vi "Calibrate In Ear (FPL).vi"(11 "State":T2) -> (0 "error out":errorcluster)   [LabVIEW 2015]
uses:
  Utility VIs/Type Defs/Speaker ring.ctl
  Utility VIs/Buttons/KCheckmarkBoolean 2.ctl
  Cochlear Function Test Suite/LV Source/CFTS Main Panel SubVIs/CFTS-Experiment State.ctl
  FPL VIs/FPL-In Ear Parameters.ctl
  FPL VIs/FPL-Stimulus.ctl
  Utility VIs/Conversion VIs/Create Waveform Cluster (2D).vi
  Utility VIs/Math VIs/FFT x(t) to dB,Degrees (2D).vi
  Instance           1 24Saved   Calibrate In Ear .vi
panel:
  in  "Start":bool
  in  "Stop":bool
  in  "FPL":T1 caption="Compute FPL"
  in  "Speaker":T3
  in  "mic gain":dbl caption="Mic Gain (dB)"
  in  "Stimulus":T4={"Resolution (Hz)"=50.0, "Attenuation (dB)"=30.0, "Sampling rate (Hz)"=100000.0}
  out "Stimulus graph":cluster{i32, dbl, dbl[]}(graph)={0, 0.01, []}
  in  "Averages":i32=128
  in  "Tabs":enum32{"Live", "Data"}(tab)
  out "Mic signals":cluster{"offset":dbl, "dx":dbl, "Y":dbl[][]}(graph)
  out "Mic mag":cluster{"offset":dbl, "dx":dbl, "Y":dbl[][]}(graph)
  out "Acquired":i32=256
  in  "Clear":bool
  in  "Load":bool
  in  "Show all":bool
  out "ASTF":cluster{"Frequency":dbl[], "Frequency":dbl[]}[](graph)
  in  "Plot Max SPL":T1=TRUE
  in  "result":cluster{"Path":path, "error ":errorcluster}
  out "Path":path
  out "ASTF phase":cluster{"Frequency":dbl[], "Frequency":dbl[]}[](graph)
  out "Mic phase graph":cluster{"offset":dbl, "dx":dbl, "Y":dbl[][]}(graph)
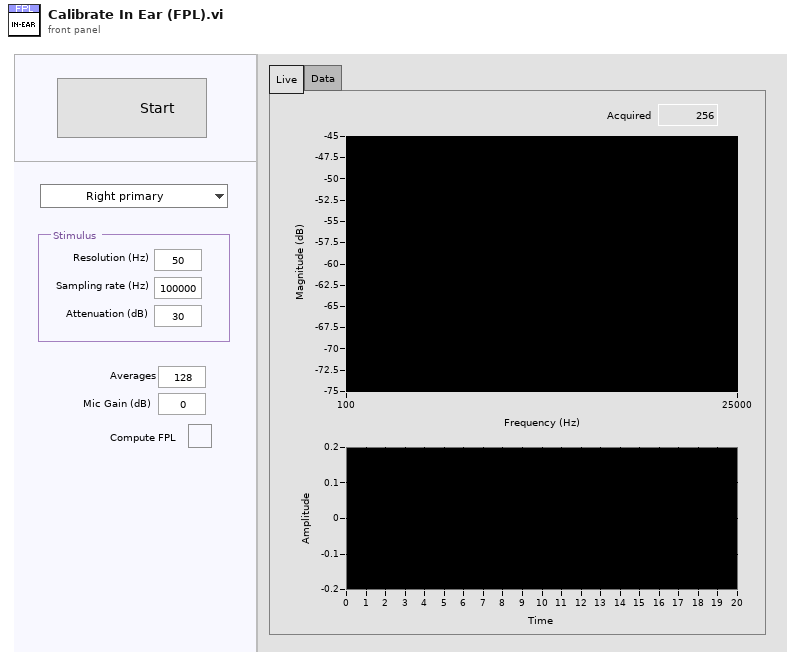
[diagram p1: front panel]
types:
  T1 = typedef "KCheckmarkBoolean 2.ctl" = bool
  T2 = typedef "CFTS-Experiment State.ctl" = cluster{"Experimenter":string, "Number":u32, "Right":string, "Left":string, "Data Folder":path, "State File":path, "Version Info":string, "End Exposure Time":dbl, "Exposure Duration":string, "Run #":cluster{"CAP":i16, "ABR":i16, "DP":i16, "VsEP":i16, "MeasSeq":i16, "SubSeq":i16, "SFOAE":i16}}
  T3 = typedef "Speaker ring.ctl" = enum16{"Right primary", "Right secondary", "Left primary", "Left secondary"}
  T4 = cluster{"Resolution (Hz)":dbl, "Attenuation (dB)":dbl, "Sampling rate (Hz)":dbl}
  T5 = typedef "FPL-In Ear Parameters.ctl" = cluster{"Speaker":T3, "Stimulus":T6, "Averages":i32, "Left gain":dbl, "Right gain":dbl, "plot max":bool, "FPL":bool}
  T6 = typedef "FPL-Stimulus.ctl" = cluster{"Resol (Hz)":dbl, "Atten (dB)":dbl, "Fs (Hz)":dbl}
  T7 = typedef "Cal Stimulus.ctl" = cluster{"Min Freq (Hz)":dbl, "Max Freq (Hz)":dbl, "Freq Step (Hz)":dbl, "Waveform":enum16{"Chirp", "Weighted"}, "Attenuation (dB)":dbl, "Sample Rate (Hz)":dbl}
  T8 = cluster{"path out":path, "error out":errorcluster}
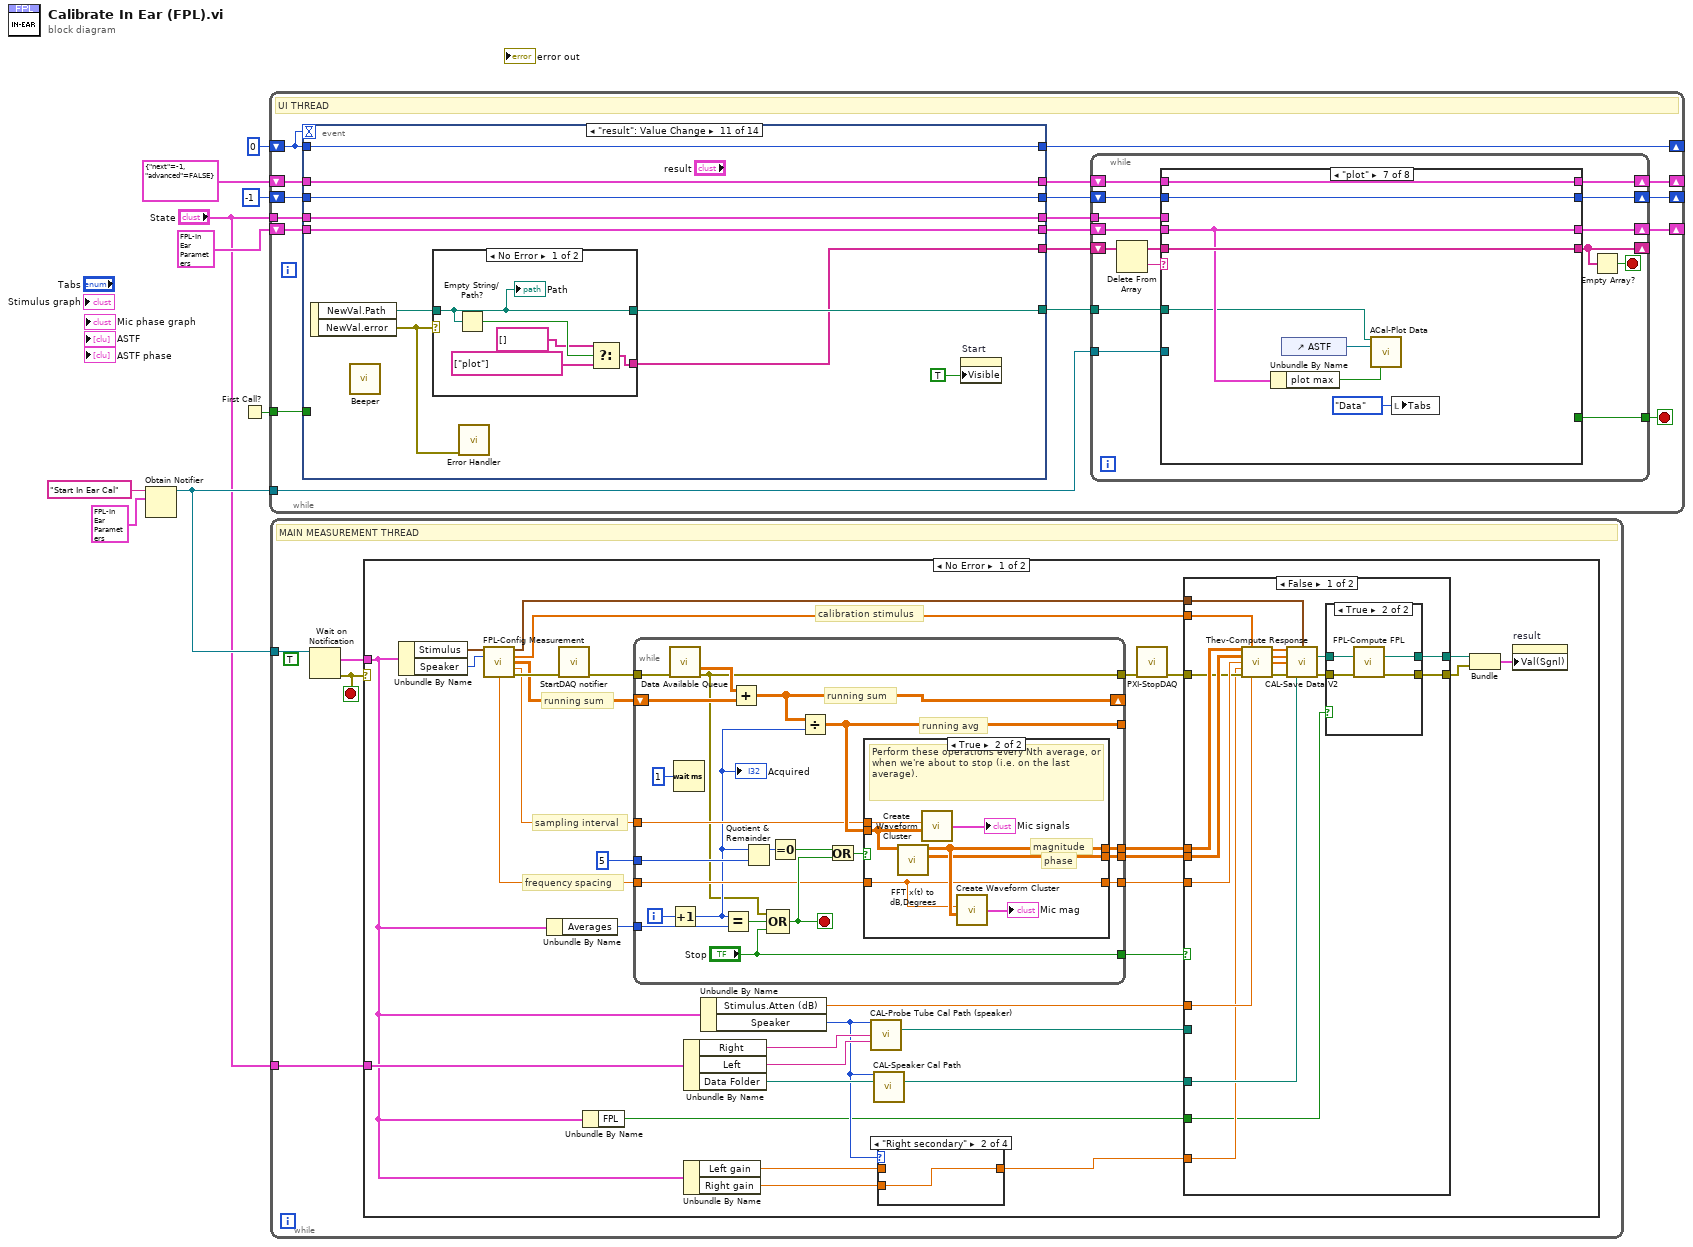
[diagram p0: block diagram]
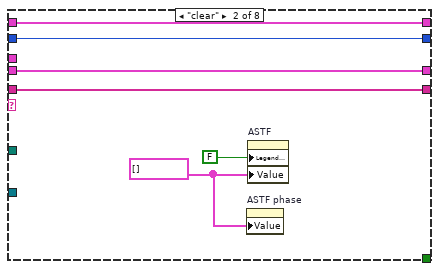
[diagram p10: hidden frame]
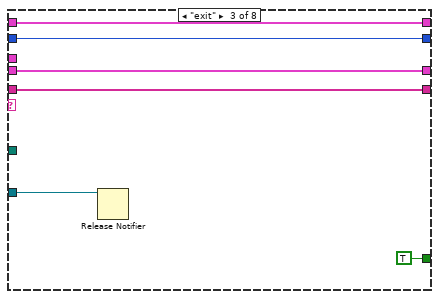
[diagram p11: hidden frame]
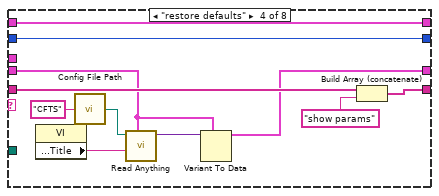
[diagram p12: hidden frame]
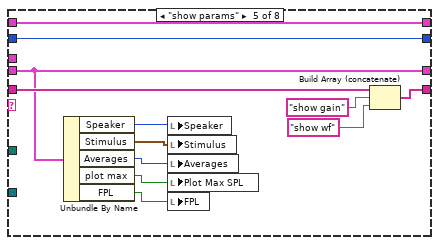
[diagram p13: hidden frame]
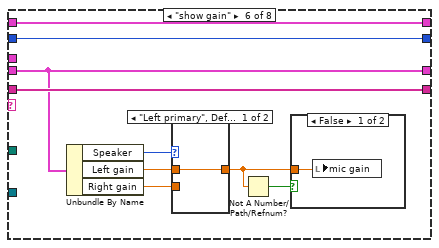
[diagram p14: hidden frame]
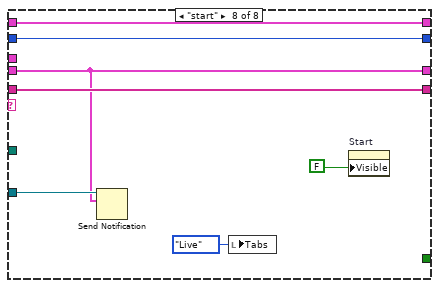
[diagram p17: hidden frame]
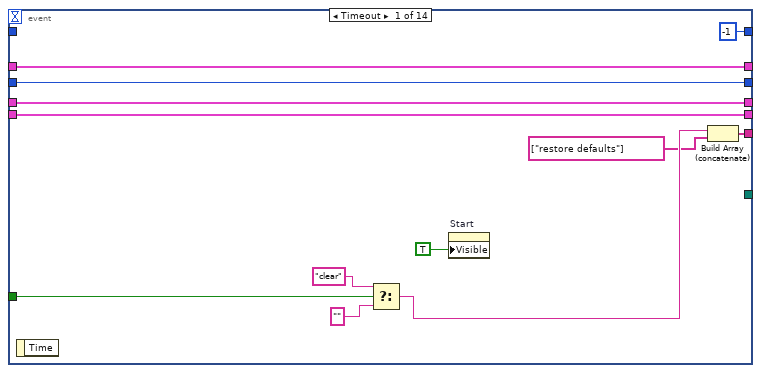
[diagram p18: hidden frame]
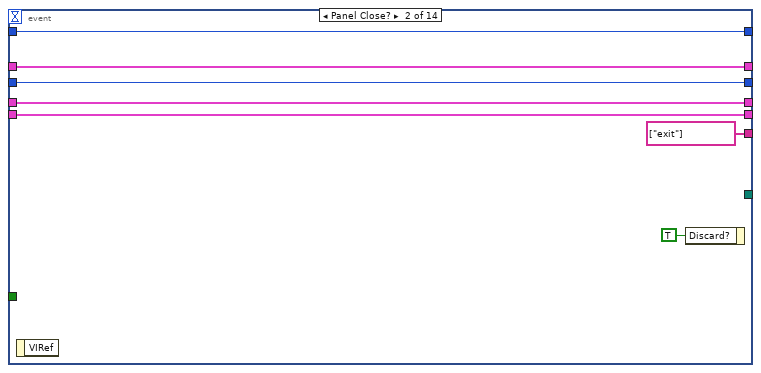
[diagram p19: hidden frame]
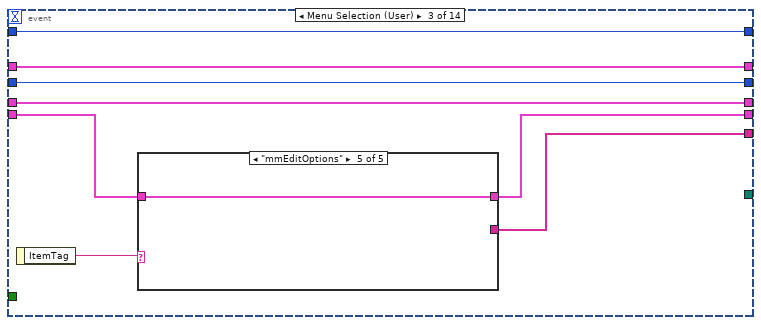
[diagram p20: hidden frame]
diagram:
  n1 = Obtain Notifier(name (unnamed)="Start In Ear Cal", notification data type=T5 {"Speaker"=enum."Right primary", "Stimulus"={"Resol (Hz)"=50.0, "Atten (dB)"=50000.0, "Fs (Hz)"=50.0}, "Averages"=512, "Left gain"=40.0, "Right gain"=40.0, "plot max"=TRUE, "FPL"=FALSE} ("Params")) -> (notifier out=w9:refnum<notifier>)  [unwired: 2 in, 2 out]
  n2 = First Call?() -> (First Call?: T/F=w1:bool)
  n3 = while {
    tunnel: w9 -> [w16]
    shift-right: [w25] -> _
    shift-left: 0 -> [w26]
    shift-right: [w19] -> _
    shift-left: -1 -> [w27]
    tunnel: "State" -> [w24]
    shift-right: [w20] -> _
    shift-left: T5 {"Speaker"=enum."Right primary", "Stimulus"={"Resol (Hz)"=50.0, "Atten (dB)"=50000.0, "Fs (Hz)"=50.0}, "Averages"=512, "Left gain"=40.0, "Right gain"=40.0, "plot max"=TRUE, "FPL"=TRUE} ("Params") -> [w23]
    shift-right: [w11] -> _
    shift-left: cluster{"next":i32, "advanced":bool} {"next"=-1, "advanced"=FALSE} -> [w13]
    tunnel: w1 -> [w10]
    stop <- w17 stop-if-true
    # "UI THREAD"
    n4 = event shown="[10] \"result\": Value Change" {
      selector: _ -> [_ _ _ _ _ _ _ _ _ _ _ _ _ _]
      dyn-events: _ -> [_ _ _ _ _ _ _ _ _ _ _ _ _ _]
      timeout: w26 -> [_ _ _ _ _ _ _ _ _ _ _ _ _ _]
      tunnel: w27 -> [w119 w126 w135 w154 w162 w165 w172 w180 w192 w205 w227 w239 w246 w261]
      tunnel: [w119 w126 w135 w154 w162 w165 w172 w180 w192 w205 w227 w239 w246 w261] -> w22
      tunnel: w26 -> [_ w125 w134 w153 w161 w170 w177 w184 w191 w204 w226 w238 w245 w259]
      tunnel: [-1 w125 w134 w153 w161 w170 w177 w184 w191 w204 w226 w238 w245 w259] -> w25
      tunnel: w24 -> [w115 w122 w129 w152 w156 w168 w175 w182 w187 w202 w224 w235 w243 w258]
      tunnel: w23 -> [w117 w124 w132 w151 w160 w169 w176 w183 w189 w203 w225 w237 w244 w257]
      tunnel: [w117 w124 w131 w151 w158 w167 w174 w181 w188 w201 w225 w237 w244 w257] -> w21
      tunnel: [w114 string[] ["exit"] w130 string[] ["start"] string[] ["show gain"] string[] ["show wf"] _ _ _ _ w219 string[] ["clear"] w241 _] -> w18
      tunnel: [w115 w122 w129 w152 w156 w168 w175 w182 w187 w202 w224 w235 w243 w258] -> w15
      tunnel: [_ _ _ _ _ _ _ _ _ _ w222 _ w242 _] -> w14
      tunnel: w13 -> [w112 w121 w128 w150 w155 w164 w171 w179 w185 w199 w221 w234 w240 w255]
      tunnel: [w112 w121 w128 w150 w155 w164 w171 w179 w185 w199 w221 w234 w240 w255] -> w12
      tunnel: w10 -> [w111 _ _ _ _ _ _ _ _ _ _ _ _ _]
      event Timeout {
        n5 = event-data() -> ()  [unwired: 1 in, 1 out]
        n6 = Select(t="clear", s=w111, f="") -> (s? t:f=w116:string)
        n7 = property on="Start" class="Bool"("Visible"=TRUE) -> ()  [unwired: 2 in, 2 out]
        n8 = Build Array (concatenate)(w116, string[] ["restore defaults"]) -> (w114:string[])
      }
      event Panel Close? {
        n9 = event-data() -> ()  [unwired: 1 in, 1 out]
        n10 = event-data("Discard?"=TRUE) -> ()  [unwired: 1 in, 1 out]
      }
      event Menu Selection (User) {
        n11 = event-data() -> ("ItemTag"=w133:string)  [unwired: 1 in]
        n12 = case shown="\"mmEditOptions\"" w133 {
          tunnel: w132 -> [w136 w138 w141 w147 w148]
          tunnel: [w136 w138 w141 w147 w148] -> w131
          tunnel: [_ string[] ["restore defaults"] _ string[] ["exit"] _] -> w130
          frame "", Default {
          }
          frame "mmFileRestore" {
          }
          frame "mmFileSave" {
            n13 = property class="VI"() -> ("Front Panel.Title"=w140:string)  [unwired: 2 in, 2 out]
            n14 = call "Config File Path.vi"("AppName"="CFTS") -> ("Default config file name"=w142:path)
            n15 = call "Write Anything.vi"("Section Name (Name of \"Anything\")"=w140, "Anything"=w141, "Path (dialog)"=w142) -> ("Error Out"=w139:errorcluster)  [unwired: 7 in, 1 out]
            n16 = case shown="Error" w139 {
              selector: w139 -> [_ w145]
              frame No Error {
                n17 = One Button Dialog(message="Defaults saved.") -> ()  [unwired: 1 in, 1 out]
              }
              frame Error {
                n18 = call "Error Handler.vi"("error in (no error)"=w145) -> ()  [unwired: 13 in, 2 out]
              }
            }
          }
          frame "mmFileExit" {
          }
          frame "mmEditOptions" {
          }
        }
      }
      event "Start": Value Change {
        n19 = event-data() -> ()  [unwired: 1 in, 1 out]
      }
      event Value Change {
        n20 = event-data() -> ("NewVal"=w157:T3)  [unwired: 1 in]
        n21 = Bundle By Name(cluster=w160, "Speaker"=w157) -> (w158:T5)
      }
      event "Stimulus": Value Change {
        n22 = event-data() -> ()  [unwired: 1 in, 1 out]
        n23 = Bundle By Name(cluster=w169, "Stimulus"="Stimulus") -> (w167:T5)
      }
      event "Averages": Value Change {
        n24 = event-data() -> ()  [unwired: 1 in, 1 out]
        n25 = Bundle By Name(cluster=w176, "Averages"="Averages") -> (w174:T5)
      }
      event Value Change {
        n26 = event-data() -> ()  [unwired: 1 in, 1 out]
        n27 = Bundle By Name(cluster=w183, "FPL"="FPL") -> (w181:T5)
      }
      event "mic gain": Value Change {
        n28 = event-data() -> ()  [unwired: 1 in, 1 out]
        n29 = Unbundle By Name(w189) -> ("Speaker"=w190:T3)
        n30 = case shown="\"Right primary\", \"Right secondary\"" w190 {
          tunnel: w189 -> [w195 w198]
          tunnel: [w194 w197] -> w188
          tunnel: "mic gain" -> [w193 w196]
          frame "Left primary", Default {
            n31 = Bundle By Name(cluster=w195, "Left gain"=w193) -> (w194:T5)
          }
          frame "Right primary", "Right secondary" {
            n32 = Bundle By Name(cluster=w198, "Right gain"=w196) -> (w197:T5)
          }
        }
      }
      event Value Change {
        # "Clear the plot because the scaling is no longer consistent with the option. We haven't retained a list of displayed data files, so we can't restore them with the proper scaling. The best we can do (without more serious revision) is to reload the last saved calibration file."
        n33 = event-data() -> ("NewVal"=w210:T1)  [unwired: 1 in]
        n34 = control-ref of="ASTF"() -> (w208:refnum<vi>)
        n35 = property class="XYGraph (strict)"(reference=w208, "Value"=cluster{"Frequency":dbl[], "Frequency":dbl[]}[] []) -> (reference out=w206:refnum<vi>, error out=w209:errorcluster)  [unwired: 1 in]
        n36 = Bundle By Name(cluster=w203, "plot max"="Plot Max SPL") -> (w201:T5)
        n37 = local read "Path"() -> (w212:path)
        n38 = call "FileIO-File or Folder Exists.vi"("error in (no error)"=w209, "path"=w212) -> ("Directory?"=w213:bool, "dup path"=w211:path)  [unwired: 6 in, 2 out]
        n39 = case shown="True" w213 {
          tunnel: w206 -> [_ w216]
          tunnel: w210 -> [_ w214]
          tunnel: w211 -> [_ w217]
          frame False {
          }
          frame True {
            n40 = call "ACal-Plot Data.vi"("Path"=w217, "Mag graph"=w216, "Plot max"=w214) -> ("error out"=w215:errorcluster)  [unwired: 11 in, 1 out]
            n41 = call <vilib>:"Simple Error Handler.vi"("error in (no error)"=w215) -> ()  [unwired: 4 in, 5 out]
          }
        }
      }
      event "result": Value Change {
        n42 = event-data() -> ("NewVal.Path"=w223:path, "NewVal.error"=w218:errorcluster)  [unwired: 1 in]
        n43 = call "Beeper.vi"() -> ()  [unwired: 5 in, 1 out]
        n44 = case shown="No Error" w218 {
          selector: w218 -> [_ w233]
          tunnel: w223 -> [w232 _]
          tunnel: [w232 _] -> w222
          tunnel: [w229 _] -> w219
          frame No Error {
            n45 = Empty String/Path?(string/path=w232) -> (empty?=w231:bool)
            n46 = Select(t=string[] [], s=w231, f=string[] ["plot"]) -> (s? t:f=w229:string[])
            "Path" <- w232
          }
          frame Error {
            n47 = call "Error Handler.vi"("error in (no error)"=w233) -> ()  [unwired: 13 in, 2 out]
          }
        }
        n48 = call "Error Handler.vi"("error in (no error)"=w218) -> ()  [unwired: 13 in, 2 out]
        n49 = property on="Start" class="Bool"("Visible"=TRUE) -> ()  [unwired: 2 in, 2 out]
      }
      event "Clear": Value Change {
        n50 = event-data() -> ()  [unwired: 1 in, 1 out]
      }
      event "Load": Value Change {
        n51 = event-data() -> ()  [unwired: 1 in, 1 out]
        n52 = Unbundle By Name(w243) -> ("Data Folder"=w247:path)
        n53 = call "File Dialog"("start path"=w247, "pattern (all files)"="*.calib", "pattern label"="Calibration files") -> ("selected path"=w252:path, "cancelled"=w251:bool, "error out"=w250:errorcluster)  [unwired: 9 in, 1 out]
        n54 = case shown="False" w251 {
          tunnel: w252 -> [w254 _]
          tunnel: w250 -> [_ _]
          tunnel: [w254 _] -> w242
          tunnel: [string[] ["plot"] _] -> w241
          frame False {
          }
          frame True {
          }
        }
      }
      event "Show all": Value Change {
        n55 = event-data() -> ()  [unwired: 1 in, 1 out]
        n56 = Unbundle By Name(w257) -> ("plot max"=w256:bool)
        n57 = Unbundle By Name(w258) -> ("Data Folder"=w262:path)
        n58 = control-ref of="ASTF"() -> (w260:refnum<vi>)
        n59 = call "CAL-Show all.vi"("Path"=w262, "Mag graph"=w260, "Plot Max SPL"=w256) -> ("error out"=w263:errorcluster)  [unwired: 11 in, 1 out]
        n60 = call "Error Handler.vi"("error in (no error)"=w263) -> ()  [unwired: 13 in, 2 out]
      }
    }
    n61 = while {
      shift-right: [w40] -> w20
      shift-left: w21 -> [w41]
      shift-right: [w39] -> w19
      shift-left: w22 -> [w42]
      shift-right: [w35] -> _
      shift-left: w18 -> [w37]
      tunnel: w16 -> [w33]
      tunnel: [w32] -> w17
      tunnel: w15 -> [w31]
      tunnel: w14 -> [w30]
      shift-right: [w29] -> w11
      shift-left: w12 -> [w28]
      stop <- w34 stop-if-true
      n62 = Delete From Array(array=w37) -> (deleted portion=w36:string, array with subset deleted=w38:string[])  [unwired: 2 in]
      n63 = case shown="\"plot\"" w36 {
        tunnel: w42 -> [w46 w52 w58 w69 w81 w90 w101 w108]
        tunnel: [w46 w52 w58 w69 w81 w90 w101 w108] -> w39
        tunnel: w41 -> [w45 w51 w57 w65 w79 w88 w99 w104]
        tunnel: [w45 w51 w57 w64 w79 w88 w99 w104] -> w40
        tunnel: w38 -> [w44 w50 w56 w68 w80 w89 w100 w105]
        tunnel: [w44 w50 w56 w63 w74 w89 w100 w105] -> w35
        tunnel: w33 -> [_ _ w55 _ _ _ _ w106]
        tunnel: [_ _ TRUE _ _ _ _ _] -> w32
        tunnel: w31 -> [_ _ _ _ _ _ _ _]
        tunnel: w30 -> [_ _ _ _ _ _ w96 _]
        tunnel: [w43 w47 w53 w59 w72 w82 w95 w107] -> w29
        tunnel: w28 -> [w43 w47 w53 w59 w72 w82 w95 w107]
        frame "", Default {
        }
        frame "clear" {
          w49 = cluster{"Frequency":dbl[], "Frequency":dbl[]}[] [] ("ASTF mag")
          n64 = property on="ASTF phase" class="XYGraph (strict)"("Value"=w49) -> ()  [unwired: 2 in, 2 out]
          n65 = property on="ASTF" class="XYGraph (strict)"("Legend Visible"=FALSE ("Legend:Visible"), "Value"=w49) -> ()  [unwired: 2 in, 2 out]
        }
        frame "exit" {
          n66 = Release Notifier(notifier=w55) -> ()  [unwired: 2 in, 3 out]
        }
        frame "restore defaults" {
          n67 = property class="VI"() -> ("Front Panel.Title"=w61:string)  [unwired: 2 in, 2 out]
          n68 = call "Config File Path.vi"("AppName"="CFTS") -> ("Default config file name"=w60:path)
          n69 = call "Read Anything.vi"("Type of Anything"=w65, "Section Name (Name of \"Type of Anything\")"=w61, "Path (dialog)"=w60) -> ("Anything"=w66:variant)  [unwired: 6 in, 2 out]
          n70 = Variant To Data(type=w65, Variant=w66) -> (data=w64:T5)  [unwired: 1 in, 1 out]
          n71 = Build Array (concatenate)(w68, "show params") -> (w63:string[])
        }
        frame "show params" {
          n72 = Unbundle By Name(w79) -> ("Speaker"=w78:T3, "Stimulus"=w77:T6, "Averages"=w76:i32, "plot max"=w75:bool, "FPL"=w70:bool)
          n73 = local write "Speaker"(w78) -> ()
          n74 = local write "Stimulus"(w77) -> ()
          n75 = local write "Averages"(w76) -> ()
          n76 = local write "Plot Max SPL"(w75) -> ()
          n77 = local write "FPL"(w70) -> ()
          n78 = Build Array (concatenate)(w80, "show gain", "show wf") -> (w74:string[])
        }
        frame "show gain" {
          n79 = Unbundle By Name(w88) -> ("Speaker"=w85:T3, "Left gain"=w84:dbl, "Right gain"=w83:dbl)
          n80 = case shown="\"Left primary\", Default" w85 {
            tunnel: w84 -> [w92 _]
            tunnel: w83 -> [_ w93]
            tunnel: [w92 w93] -> w87
            frame "Left primary", Default {
            }
            frame "Right primary", "Right secondary" {
            }
          }
          n81 = Not A Number/Path/Refnum?(number/path/refnum=w87) -> (NaN/Path/Refnum?=w86:bool)
          n82 = case shown="False" w86 {
            tunnel: w87 -> [w91 _]
            frame False {
              n83 = local write "mic gain"(w91) -> ()
            }
            frame True {
            }
          }
        }
        frame "plot" {
          n84 = Unbundle By Name(w99) -> ("plot max"=w98:bool)
          n85 = control-ref of="ASTF"() -> (w97:refnum<vi>)
          n86 = call "ACal-Plot Data.vi"("Path"=w96, "Mag graph"=w97, "Plot max"=w98) -> ()  [unwired: 11 in, 2 out]
          n87 = local write "Tabs"(enum32{"Live", "Data"}."Data" ("Tabs")) -> ()
        }
        frame "start" {
          n88 = Send Notification(notification=w104, notifier=w106) -> ()  [unwired: 1 in, 2 out]
          n89 = local write "Tabs"(enum32{"Live", "Data"}."Live" ("Tabs")) -> ()
          n90 = property on="Start" class="Bool"("Visible"=FALSE) -> ()  [unwired: 2 in, 2 out]
        }
      }
      n91 = Empty Array?(array=w35) -> (empty?=w34:bool)
    }
  }
  n92 = while {
    tunnel: w9 -> [w267]
    tunnel: "State" -> [w265]
    stop <- w266 stop-if-true
    (unwired) TRUE
    # "MAIN MEASUREMENT THREAD"
    n93 = Wait on Notification(notifier=w267) -> (notification=w264:T5, error out=w266:errorcluster)  [unwired: 3 in, 2 out]
    n94 = case shown="No Error" w266 {
      tunnel: w265 -> [w282 _]
      tunnel: w264 -> [w270 _]
      frame No Error {
        # "calibration stimulus"
        # "frequency spacing"
        # "sampling interval"
        # "running sum"
        n95 = Unbundle By Name(w270) -> ("Stimulus"=w268:T6, "Speaker"=w281:T3)
        n96 = call "FPL-Config Measurement.vi"("Chirp spec in"=w268, "Speaker"=w281) -> ("Cal Stimulus"=w284:T7, "Stimulus"=w293:dbl[], "Mic Avg"=w299:dbl[][], "dt (ms)"=w297:dbl, "df (Hz)"=w298:dbl, "error out"=w300:errorcluster)  [unwired: 8 in]
        n97 = Unbundle By Name(w270) -> ("Averages"=w280:i32)
        n98 = call "StartDAQ notifier.vi"("error in (no error)"=w300) -> ("error out"=w292:errorcluster)  [unwired: 6 in]
        n99 = Unbundle By Name(w270) -> ("FPL"=w269:bool)
        n100 = while {
          tunnel: w292 -> [w351]
          tunnel: [w331] -> w291
          tunnel: w280 -> [w348]
          shift-right: [w346] -> _
          shift-left: w299 -> [w347]
          tunnel: [w345] -> _
          tunnel: 5 -> [w344]
          tunnel: w298 -> [w339]
          tunnel: [w338] -> w296
          tunnel: [w337] -> w295
          tunnel: w297 -> [w336]
          tunnel: [w335] -> w294
          tunnel: ["Stop"] -> w278
          i -> [w350]
          stop <- w340 stop-if-true
          # "running avg"
          # "running sum"
          n101 = call "Data Available Queue.vi"("error in (no error)"=w351) -> ("AI Waveforms"=w333:dbl[][], "error out"=w331:errorcluster)  [unwired: 10 in, 3 out]
          n102 = Increment(x=w350) -> (x+1=w334:i32)
          "Acquired" <- w334
          n103 = Wait (ms)(milliseconds to wait=u32 1) -> ()  [unwired: 1 out]
          n104 = Equal?(x=w334, y=w348) -> (x = y?=w349:bool)
          n105 = Add(x=w333, y=w347) -> (x+y=w346:dbl[][])
          n106 = Quotient & Remainder(x=w334, y=w344) -> (x-y*floor(x/y)=w343:i32)  [unwired: 1 out]
          n107 = Compound Arithmetic op=OR(w331, w349, "Stop") -> (w340:bool)
          n108 = Equal To 0?(x=w343) -> (x = 0?=w341:bool)
          n109 = Divide(x=w346, y=w334) -> (x/y=w345:dbl[][])
          n110 = Or(x=w341, y=w340) -> (x .or. y?=w342:bool)
          n111 = case shown="True" w342 {
            tunnel: w345 -> [_ w355]
            tunnel: w339 -> [_ w352]
            tunnel: [_ w357] -> w338
            tunnel: [_ w356] -> w337
            tunnel: w336 -> [_ w354]
            tunnel: [_ w352] -> w335
            frame False {
            }
            frame True {
              # "phase"
              # "magnitude"
              # "Perform these operations every Nth average, or when we're about to stop (i.e. on the last average)."
              n112 = call-poly "FFT x(t) to dB,Degrees.vi"("X(t)"=w355) -> ("+Freq Phase of FFT (degrees)"=w356:dbl[][], "+Freq. Mag of FFT (dB rms)"=w357:dbl[][])  [unwired: 9 in]
              n113 = call-poly "Create Waveform Cluster.vi"("dx"=w354, "Array"=w355) -> ("waveform cluster"=→"Mic signals":cluster{"offset":dbl, "dx":dbl, "Y":dbl[][]})  [unwired: 3 in]
              n114 = call-poly "Create Waveform Cluster.vi"("dx"=w352, "Array"=w357) -> ("waveform cluster"=→"Mic mag":cluster{"offset":dbl, "dx":dbl, "Y":dbl[][]})  [unwired: 3 in]
            }
          }
        }
        n115 = Unbundle By Name(w282) -> ("Right"=w289:string, "Left"=w288:string, "Data Folder"=w287:path)
        n116 = Unbundle By Name(w270) -> ("Left gain"=w276:dbl, "Right gain"=w274:dbl)
        n117 = Unbundle By Name(w270) -> ("Stimulus.Atten (dB)"=w279:dbl, "Speaker"=w277:T3)
        n118 = call "CAL-Probe Tube Cal Path (speaker).vi"("Speaker"=w277, "Right"=w289, "Left"=w288) -> ("Probe Tube Cal Path"=w286:path)  [unwired: 11 in, 1 out]
        n119 = call "CAL-Speaker Cal Path.vi"("Speaker"=w277, "Data Folder"=w287) -> ("Cal Path"=w283:path)  [unwired: 12 in, 1 out]
        n120 = case shown="\"Right secondary\"" w277 {
          tunnel: w276 -> [_ _ w303 w304]
          tunnel: [w301 w302 w303 w304] -> w275
          tunnel: w274 -> [w301 w302 _ _]
          frame "Right primary", Default {
          }
          frame "Right secondary" {
          }
          frame "Left secondary" {
          }
          frame "Left primary" {
          }
        }
        n121 = call "PXI-StopDAQ.vi"("error in (no error)"=w291) -> ("error out"=w285:errorcluster)  [unwired: 6 in]
        n122 = case shown="False" w278 {
          tunnel: w296 -> [w322 _]
          tunnel: w295 -> [w321 _]
          tunnel: w294 -> [w320 _]
          tunnel: w293 -> [w319 _]
          tunnel: w286 -> [_ _]
          tunnel: w285 -> [w318 w329]
          tunnel: w284 -> [w310 _]
          tunnel: w283 -> [w317 _]
          tunnel: w279 -> [w316 _]
          tunnel: [w306 w329] -> w272
          tunnel: [w307 _] -> w273
          tunnel: w275 -> [w315 _]
          tunnel: w269 -> [w305 _]
          frame False {
            n123 = call "Thev-Compute Response.vi"("Mag"=w322, "Stimulus"=w319, "Phase"=w321, "df (Hz)"=w320, "Probe Mic Gain (dB)"=w315, "error in (no error)"=w318, "Attenuation (dB)"=w316) -> ("ASTF Mag"=w311:dbl[], "ASTF Phase"=w312:dbl[], "Frequency"=w313:dbl[], "error out"=w314:errorcluster)  [unwired: 5 in]
            n124 = call "CAL-Save Data V2.vi"("Mag"=w311, "Cal Stimulus"=w310, "Phase"=w312, "Frequency"=w313, "error in (no error)"=w314, "path"=w317) -> ("new file path"=w308:path, "error out"=w309:errorcluster)  [unwired: 8 in]
            n125 = case shown="True" w305 {
              tunnel: w309 -> [w323 w328]
              tunnel: w308 -> [w324 w327]
              tunnel: [w324 w326] -> w307
              tunnel: [w323 w325] -> w306
              frame False {
              }
              frame True {
                n126 = call "FPL-Compute FPL.vi"("path in"=w327, "error in (no error)"=w328) -> ("path out"=w326:path, "error out"=w325:errorcluster)  [unwired: 12 in]
              }
            }
          }
          frame True {
          }
        }
        n127 = Bundle("path out"=w273, "error out"=w272) -> (w271:T8)  [unwired: 1 in]
        n128 = property on="result" class="Clust (strict)"("Val(Sgnl)"=w271) -> ()  [unwired: 2 in, 2 out]
      }
      frame Error {
      }
    }
  }
